vi "Read Sweep Configuration Example.vi"   [LabVIEW 2019, in "Sweep Control.lvclass"]
uses:
  Sweep Control.lvclass
  Typedefs/Enum - Experiments.ctl
  Typedefs/Continuous B Sweep JSON--Cluster.ctl
  Typedefs/Enum - Priority.ctl
  Typedefs/Enum - Action.ctl
  Typedefs/Cluster - ScanControl.ctl
  Typedefs/ScanControl.ctl
  Typedefs/Cluster - ScanParamters.ctl
  Typedefs/ScanParamters.ctl
  Typedefs/Sweep Control JSON--Cluster.ctl
  <userlib>/LevyLab/Transport/Transport/Typedefs/Lockin_Sweep JSON--Cluster.ctl
  <userlib>/LevyLab/Transport/Transport/Transport.lvclass
  <userlib>/LevyLab/Transport/Control Experiment/Typedefs/Wiring Description--cluster.ctl
  <userlib>/LevyLab/Transport/Control Experiment/Control Experiment.lvclass
  <userlib>/LevyLab/Transport/Control Experiment/Typedefs/Instrument--enum.ctl
  <userlib>/LevyLab/Transport/Control Experiment/Typedefs/Experiment Description--cluster.ctl
  <userlib>/LevyLab/Transport/Control Experiment/Typedefs/Instrument Types--combo.ctl
  <userlib>/LevyLab/Lockin-Multichannel/Instrument.DAQ/Typedefs/REF.Channel--Cluster--Array.ctl
  <userlib>/LevyLab/Lockin-Multichannel/Instrument.DAQ/Instrument.DAQ.lvclass
  <userlib>/LevyLab/Lockin-Multichannel/Instrument.DAQ/Typedefs/AO.Channel--Cluster--Array.ctl
  <userlib>/LevyLab/Lockin-Multichannel/Instrument.DAQ/Typedefs/Sweep.Pattern--Enum.ctl
  <userlib>/LevyLab/Transport/Control Experiment/Typedefs/Instruments--cluster.ctl
  <userlib>/LevyLab/Krohn Hite 7008/KH7008/typedefs/Filter--Enum.ctl
  <userlib>/LevyLab/Krohn Hite 7008/KH7008/KH7008.lvlib
  <userlib>/LevyLab/Krohn Hite 7008/KH7008/typedefs/couple--Enum.ctl
  <userlib>/LevyLab/Krohn Hite 7008/KH7008/typedefs/shunt--enum.ctl
  <userlib>/LevyLab/Krohn Hite 7008/KH7008/typedefs/Input--Enum.ctl
  <userlib>/LevyLab/Krohn Hite 7008/KH7008/typedefs/gain--enum.ctl
  <userlib>/LevyLab/Krohn Hite 7008/KH7008/typedefs/channel--numeric.ctl
  <userlib>/LevyLab/Krohn Hite 7008/KH7008/typedefs/channelProperties--Cluster.ctl
  <userlib>/LevyLab/Krohn Hite 7008/KH7008/typedefs/allChannelProperties--Array.ctl
  <userlib>/LevyLab/Lockin-Multichannel/Instrument.DAQ/Typedefs/AO.Channel.Function--Enum.ctl
  <userlib>/LevyLab/Lockin-Multichannel/Instrument.DAQ/Typedefs/AO.Channel--Cluster.ctl
  <userlib>/LevyLab/Lockin-Multichannel/Instrument.DAQ/Typedefs/REF.Channel--Cluster.ctl
  <userlib>/LevyLab/Lockin-Multichannel/Instrument.DAQ/Typedefs/Sweep.Channel--Cluster.ctl
  <userlib>/LevyLab/Lockin-Multichannel/Instrument.DAQ/Typedefs/Sweep.Channel--Cluster--Array.ctl
panel:
  # "See block diagram for example of how to use ReadSweepConfigurationFile.vi"
types:
  T1 = typedef "Transport.lvclass/Lockin_Sweep JSON--Cluster.ctl" = cluster{"Sweep Time (s)":dbl, "Initial Wait (s)":dbl, "Return to Start":bool, "Sweep Channels":T2, "Sweep Tables":cluster{"Ch":i32, "Table":dbl[]}[]}
  T2 = typedef "Instrument.Lockin.lvlib/Instrument.DAQ.lvclass/Sweep.Channel--Cluster--Array.ctl" = T3[]
  T3 = typedef "Instrument.Lockin.lvlib/Instrument.DAQ.lvclass/Sweep.Channel--Cluster.ctl" = cluster{"Enable?":bool, "Channel":u16, "Start":dbl, "End":dbl, "Pattern":T4, "Table":dbl[]}
  T4 = typedef "Instrument.Lockin.lvlib/Instrument.DAQ.lvclass/Sweep.Pattern--Enum.ctl" = enum16{"Ramp /", "Ramp /\\", "Smooth Ramp _/", "Smooth Ramp _/\\_", "Table"}
  T5 = typedef "Sweep Control.lvclass/Sweep Control JSON--Cluster.ctl" = cluster{"Experiment":T6, "Repeat Experiment":i32, "Scan control":T7, "Scan parameters":T11}
  T6 = typedef "Sweep Control.lvclass/Enum - Experiments.ctl" = enum16{"Lockin_time", "Lockin_sweep", "Lockin_DelayLine"}
  T7 = typedef "Sweep Control.lvclass/ScanControl.ctl" = T8[]
  T8 = typedef "Sweep Control.lvclass/Cluster - ScanControl.ctl" = cluster{"Priority":T9, "Scan name":T10}
  T9 = typedef "Sweep Control.lvclass/Enum - Priority.ctl" = enum16{"Priority 0", "Priority 1", "Priority 2", "Priority 3", "Priority 4", "Priority 5"}
  T10 = typedef "Sweep Control.lvclass/Enum - Action.ctl" = enum16{"OFF", "time", "Lockin Amplitude", "Lockin Frequency", "Lockin Bias", "Delay", "Strain", "DAQ Bias", "Magnet Field", "Temperature", "MW f1", "MW f2", "MW Amplitude1", "MW Amplitude2"}
  T11 = typedef "Sweep Control.lvclass/ScanParamters.ctl" = T12[]
  T12 = typedef "Sweep Control.lvclass/Cluster - ScanParamters.ctl" = cluster{"Start":dbl, "End":dbl, "Step":dbl, "Rate":dbl, "Waveform type":enum16{"linear", "triangle", "power"}, "wait (ms or K)":dbl, "Address":string, "channel":i32}
  T13 = typedef "Sweep Control.lvclass/Continuous B Sweep JSON--Cluster.ctl" = cluster{"Continuous B Sweep":cluster{"Experiment":T6, "B field values":dbl[]}, "Experiment Description":T14, "Wiring Configuration":T18, "Lockin":cluster{"AOconfig":T19, "REFconfig":T22}, "Krohn Hite":cluster{"Channel Setting":T24}}
  T14 = typedef "Control Experiment.lvclass/Experiment Description--cluster.ctl" = cluster{"User":string, "Device":string, "Device Path":path, "Device Description":string, "Experiment Path":path, "Experiment Description":string, "Instrument":T15, "Instruments":T16[], "Sweep":cluster{"key":string, "value":variant}[]}
  T15 = typedef "Control Experiment.lvclass/Instrument--enum.ctl" = enum16{"----- AFM/EBL -----", "AGILENT", "CYPHER", "Gemini2", "JEOL", "MFP3D", "----- Cryostat -----", "CF900", "DR200", "MNK", "PPMS (simulated)", "PPMS 1", "PPMS 2", "PPMS 3", "----- Optics -----", "THz 1 (Element 2/Montana)", "THz 2 (Tsunami/Janis)"}
  T16 = typedef "Control Experiment.lvclass/Instruments--cluster.ctl" = cluster{"class path":path, "Address":string, "Type":T17}
  T17 = typedef "Control Experiment.lvclass/Instrument Types--combo.ctl" = string
  T18 = typedef "Control Experiment.lvclass/Wiring Description--cluster.ctl" = cluster{"Lockin Ch":i32[], "KH":cluster{"Electrodes":string[], "Labels":string[]}, "not KH":cluster{"Electrodes":string[], "Labels":string[]}}
  T19 = typedef "Instrument.Lockin.lvlib/Instrument.DAQ.lvclass/AO.Channel--Cluster--Array.ctl" = T20[]
  T20 = typedef "Instrument.Lockin.lvlib/Instrument.DAQ.lvclass/AO.Channel--Cluster.ctl" = cluster{"Enable?":bool, "Channel":i32, "Amplitude":dbl, "Offset":dbl, "Frequency":dbl, "Phase":dbl, "Function":T21, "Sweeping?":bool}
  T21 = typedef "Instrument.Lockin.lvlib/Instrument.DAQ.lvclass/AO.Channel.Function--Enum.ctl" = enum16{"Sine", "Triangle", "Square"}
  T22 = typedef "Instrument.Lockin.lvlib/Instrument.DAQ.lvclass/REF.Channel--Cluster--Array.ctl" = T23[]
  T23 = typedef "Instrument.Lockin.lvlib/Instrument.DAQ.lvclass/REF.Channel--Cluster.ctl" = cluster{"Enable?":bool, "Channel":i32, "Frequency":dbl, "Phase":dbl, "TC":dbl, "Roll-Off":i32}
  T24 = typedef "KH7008.lvlib/allChannelProperties--Array.ctl" = T25[]
  T25 = typedef "KH7008.lvlib/channelProperties--Cluster.ctl" = cluster{"channel":T26, "gain":T27, "input":T28, "shunt":T29, "couple":T30, "filter":T31}
  T26 = typedef "KH7008.lvlib/channel--numeric.ctl" = u16
  T27 = typedef "KH7008.lvlib/gain--enum.ctl" = enum16{"1", "10", "100", "1000"}
  T28 = typedef "KH7008.lvlib/Input--Enum.ctl" = enum16{"OFF", "SE+", "SE-", "DIFF"}
  T29 = typedef "KH7008.lvlib/shunt--enum.ctl" = enum16{"Open", "50", "500", "5k", "50k", "10M"}
  T30 = typedef "KH7008.lvlib/couple--Enum.ctl" = enum16{"AC", "DC"}
  T31 = typedef "KH7008.lvlib/Filter--Enum.ctl" = enum16{"OFF", "ON"}
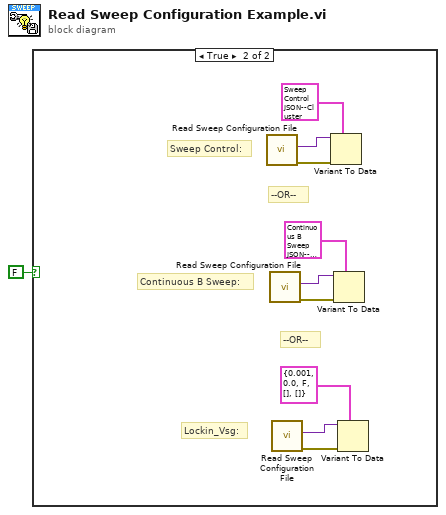
[diagram p0: block diagram]
diagram:
  n1 = case shown="True" FALSE {
    frame False {
    }
    frame True {
      # "Lockin_Vsg:"
      # "Continuous B Sweep:"
      # "Sweep Control:"
      # "--OR--"
      # "--OR--"
      n2 = call "Read Sweep Configuration File.vi"() -> ("error out"=w10:errorcluster, "Data"=w6:variant)  [unwired: 9 in, 1 out]
      n3 = call "Read Sweep Configuration File.vi"() -> ("error out"=w7:errorcluster, "Data"=w5:variant)  [unwired: 9 in, 1 out]
      n4 = call "Read Sweep Configuration File.vi"() -> ("error out"=w9:errorcluster, "Data"=w8:variant)  [unwired: 9 in, 1 out]
      n5 = Variant To Data(error in=w10, type=T5 {"Experiment"=enum."Lockin_DelayLine", "Repeat Experiment"=0, "Scan control"=[], "Scan parameters"=[]} ("SweepControl"), Variant=w6) -> ()  [unwired: 2 out]
      n6 = Variant To Data(error in=w7, type=T13 {"Continuous B Sweep"={"Experiment"=enum."Lockin_DelayLine", "B field values"=[]}, "Experiment Description"={"User"="", "Device"="", "Device Path"=path "", "Device Description"="", "Experiment Path"=path "", "Experiment Description"="", "Instrument"=enum."----- AFM/EBL -----", "Instruments"=[], "Sweep"=[]}, "Wiring Configuration"={"Lockin Ch"=[], "KH"={"Electrodes"=[], "Labels"=[]}, "not KH"={"Electrodes"=[], "Labels"=[]}}, "Lockin"={"AOconfig"=[], "REFconfig"=[]}, "Krohn Hite"={"Channel Setting"=[]}} ("ContinuousBSweep"), Variant=w5) -> ()  [unwired: 2 out]
      n7 = Variant To Data(error in=w9, type=T1 {"Sweep Time (s)"=0.001, "Initial Wait (s)"=0.0, "Return to Start"=FALSE, "Sweep Channels"=[], "Sweep Tables"=[]} ("LockinVsg Sweep"), Variant=w8) -> ()  [unwired: 2 out]
    }
  }
